vi "Read Make, Model.vi"(8 "error in (no error)":errorcluster, 11 "Camera in":refnum<class "Camera.lvclass">) -> (0 "error out":errorcluster, 2 "Make, Model":string, 3 "Camera out":refnum<class "Camera.lvclass">)   [LabVIEW 2017, in "Camera.lvclass"]
uses:
  Camera.lvclass
  Camera.lvclass/Camera.ctl
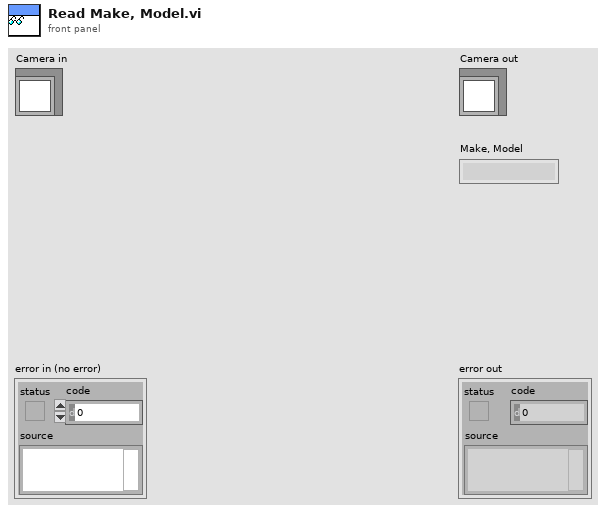
[diagram p1: front panel]
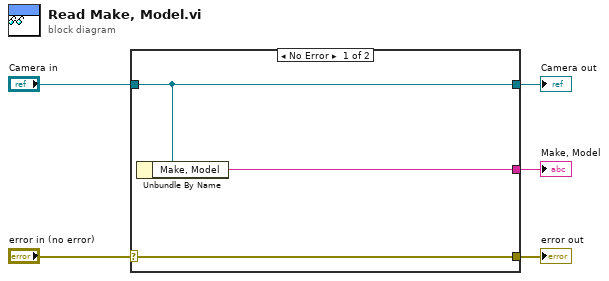
[diagram p0: block diagram]
diagram:
  n1 = case shown="No Error" "error in (no error)" {
    selector: "error in (no error)" -> [w8 w9]
    tunnel: [w8 w9] -> w4
    tunnel: [w7 w10] -> w2
    tunnel: "Camera in" -> [w7 w10]
    tunnel: [w6 _] -> w1
    frame No Error {
      n2 = Unbundle By Name(w7) -> ("Make, Model"=w6:string)
    }
    frame Error {
    }
  }
  "error out" <- w4
  "Camera out" <- w2
  "Make, Model" <- w1
